vi "Write Last Image Name.vi"(8 "error in (no error)":errorcluster, 11 "Save Image in":refnum<class "Save Image.lvclass">) -> (0 "error out":errorcluster, 3 "Save Image out":refnum<class "Save Image.lvclass">)   [LabVIEW 2018]
uses:
  Simulated_Header/Simulated_Header.lvclass
  Save Image.lvclass
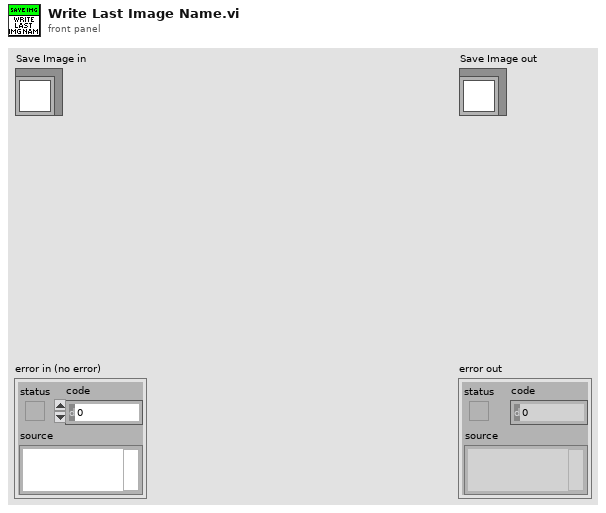
[diagram p1: front panel]
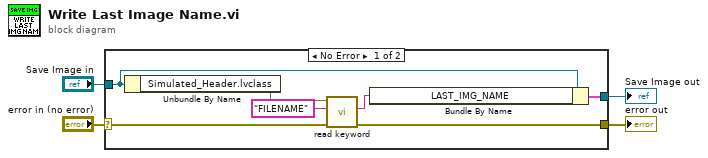
[diagram p0: block diagram]
diagram:
  n1 = case shown="No Error" "error in (no error)" {
    selector: "error in (no error)" -> [w9 w13]
    tunnel: [w8 w13] -> w3
    tunnel: [w11 w12] -> w1
    tunnel: "Save Image in" -> [w10 w12]
    frame No Error {
      n2 = Unbundle By Name(w10) -> ("Simulated_Header.lvclass"=w7)
      n3 = call "read keyword.vi"("error in (no error)"=w9, "keyword"="FILENAME", "Simulated_Header in"=w7) -> ("error out"=w8:errorcluster, "value"=w5:string)  [unwired: 6 in, 1 out]
      n4 = Bundle By Name(cluster=w10, "LAST_IMG_NAME"=w5) -> (w11:cluster{})
    }
    frame Error {
    }
  }
  "error out" <- w3
  "Save Image out" <- w1
